vi "FGV - KH Settings.vi"(4 "error in":errorcluster, 6 "Function":enum16{"write", "read"}(ring), 7 "Channel Setting":T1(array[cluster])=[{"Channel"=1, "Gain"=1, "Shunt Resistor"=1, "Measure"=2}, {"Channel"=2, "Gain"=3, "Shunt Resistor"=5, "Measure"=1}, {"Channel"=3, "Gain"=3, "Shunt Resistor"=1, "Measure"=2}, {"Channel"=4, "Gain"=4, "Shunt Resistor"=1, "Measure"=2}, {"Channel"=5, "Gain"=4, "Shunt Resistor"=1, "Measure"=2}, {"Channel"=6, "Gain"=4, "Shunt Resistor"=5, "Measure"=1}, {"Channel"=7, "Gain"=3, "Shunt Resistor"=1, "Measure"=2}, {"Channel"=8, "Gain"=3, "Shunt Resistor"=5, "Measure"=1}] {"Measure" items=["Float", "Current(Diff)", "Voltage(SE+)"]; "Shunt Resistor" items=["Open"=1, "50 Ohms"=2, "500 Ohms"=3, "5k Ohms"=4, "50k Ohms"=5]; "Gain" items=["1x"=1, "10x"=2, "100x"=3, "1000x"=4]; "Channel" items=["Channel 1"=1, "Channel 2"=2, "Channel 3"=3, "Channel 4"=4, "Channel 5"=5, "Channel 6"=6, "Channel 7"=7, "Channel 8"=8]}) -> (0 "error out":errorcluster, 3 "Channel Setting 2":T1(array[cluster]))   [LabVIEW 2013]
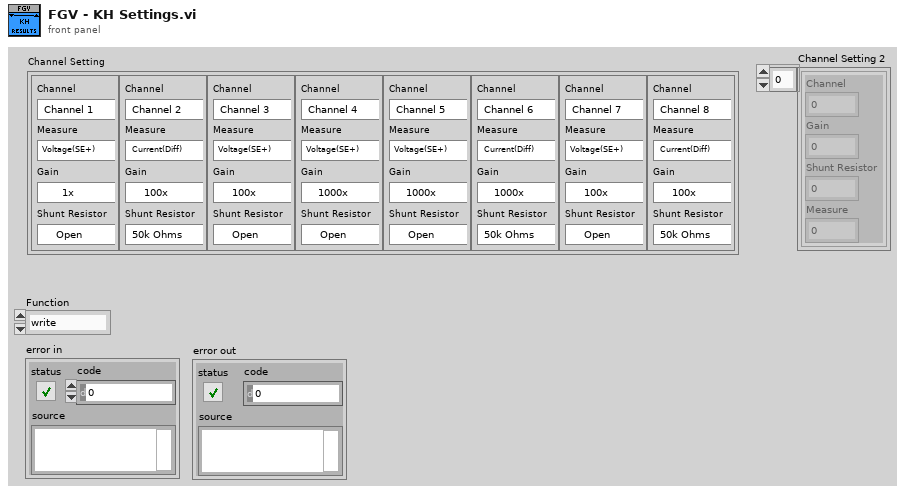
[diagram p1: front panel]
types:
  T1 = cluster{"Channel":u16, "Gain":u16, "Shunt Resistor":u16, "Measure":u16}[]
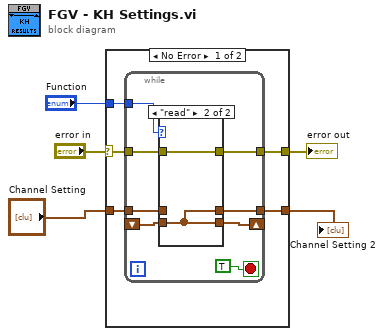
[diagram p0: block diagram]
diagram:
  n1 = case shown="No Error" "error in" {
    selector: "error in" -> [w10 w24]
    tunnel: [w9 w24] -> w4
    tunnel: "Channel Setting" -> [w8 w23]
    tunnel: [w7 w23] -> w2
    tunnel: "Function" -> [w6 _]
    frame No Error {
      n2 = while {
        shift-right: [w12] -> _
        shift-left: _ -> [w11]
        tunnel: w10 -> [w17]
        tunnel: [w16] -> w9
        tunnel: w8 -> [w15]
        tunnel: [w14] -> w7
        tunnel: w6 -> [w13]
        stop <- TRUE stop-if-true
        n3 = case shown="\"read\"" w13 {
          tunnel: w17 -> [w19 w22]
          tunnel: [w19 w22] -> w16
          tunnel: w15 -> [w20 _]
          tunnel: [w20 w21] -> w14
          tunnel: [w20 w21] -> w12
          tunnel: w11 -> [_ w21]
          frame "write", Default {
          }
          frame "read" {
          }
        }
      }
    }
    frame Error {
    }
  }
  "error out" <- w4
  "Channel Setting 2" <- w2
